vi "test Deployment Timing Channels.vi"(8 "error in":errorcluster, 11 "TestCase in":refnum<class "Deployment.lvclass">) -> (0 "error out":errorcluster, 3 "TestCase out":refnum<class "Deployment.lvclass">)   [LabVIEW 2023, in "Deployment.lvclass"]
uses:
  Deployment.lvclass
  Deployment.lvclass/Deployment.ctl
  <vilib>/addons/_JKI Toolkits/VI Tester/TestCase.llb/TestCase.lvclass
  315b1c3a-44c8-49e8-b756-01f865c29b4a.vi
  <vilib>/NI/VeriStand Custom Device Testing Tools/VeriStandTestUtilities/VeriStandTestUtilities.lvlib
  Scripting/Ballard MIL-STD-1553 Scripting.lvlib
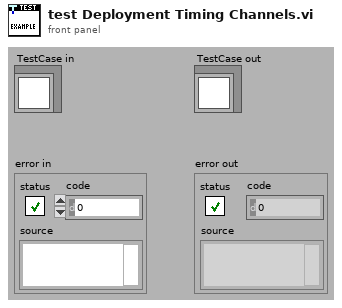
[diagram p1: front panel]
types:
  T1 = cluster{"Hardware File":path, "Parameters File":path}
  T2 = typedef "Custom Device API.lvlib/Custom Device Item Ref.ctl" = u64
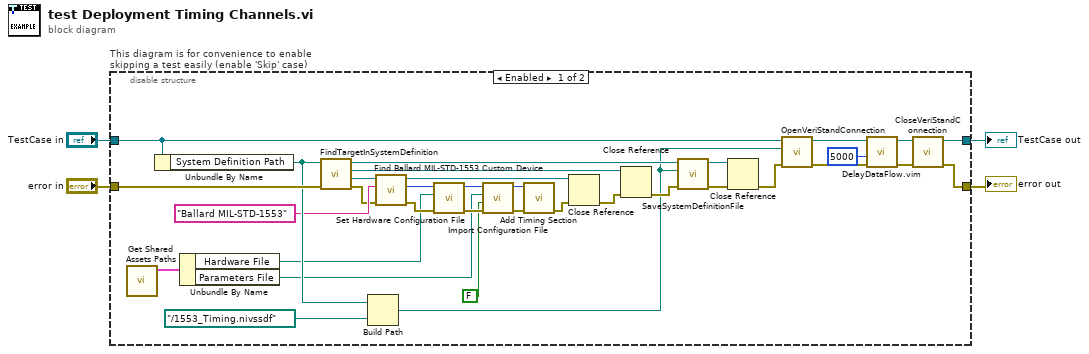
[diagram p0: block diagram]
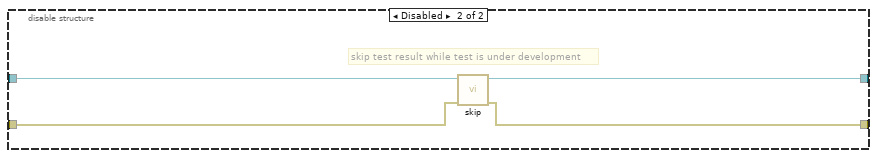
[diagram p2: hidden frame]
diagram:
  n1 = disable-structure "This diagram is for convenience to enable skipping a test easily (enable 'Skip' case)" shown="Enabled" {
    disable-tunnel: "TestCase in" -> [w31 w41]
    disable-tunnel: [w32 w39] -> w1
    disable-tunnel: [w34 w40] -> w3
    disable-tunnel: "error in" -> [w30 w38]
    frame Enabled {
      n2 = call "Get Shared Assets Paths.vi"() -> ("BC and RTs"=w8:T1)  [unwired: 9 in, 2 out]
      n3 = Unbundle By Name(w31) -> ("System Definition Path"=w28:path)
      n4 = Unbundle By Name(w8) -> ("Hardware File"=w10:path, "Parameters File"=w9:path)
      n5 = call <vilib>:"FindTargetInSystemDefinition.vi"("error in"=w30, "system definition path"=w28) -> ("error out"=w17:errorcluster, "Target"=w20:refnum<k24>, "Root"=w23:refnum<k24>, "System Definition"=w29:refnum<k24>)  [unwired: 6 in]
      n6 = Build Path(base path=w28, name or relative path=path "../1553_Timing.nivssdf") -> (appended path=w16:path)
      n7 = call "Find Ballard MIL-STD-1553 Custom Device.vi"("error in"=w17, "name"="Ballard MIL-STD-1553", "target in"=w20) -> ("error out"=w14:errorcluster, "Ballard MIL-STD 1553 custom device"=w13:T2, "target out"=w18:refnum<k24>)  [unwired: 5 in, 1 out]
      n8 = call "Set Hardware Configuration File.vi"("error in"=w14, "hardware configuration file path"=w10, "Ballard MIL-STD 1553 custom device in"=w13) -> ("error out"=w11:errorcluster, "Ballard MIL-STD 1553 custom device out"=w12:T2)  [unwired: 7 in]
      n9 = call "Import Configuration File.vi"("error in"=w11, "create Tx/Rx folders for subaddresses?"=FALSE, "parameters configuration file path"=w9, "Ballard MIL-STD 1553 custom device in"=w12) -> ("error out"=w15:errorcluster, "Ballard MIL-STD 1553 custom device out"=w6:T2)  [unwired: 6 in]
      n10 = call "Add Timing Section.vi"("error in"=w15, "custom device in"=w6) -> ("error out"=w7:errorcluster)  [unwired: 7 in, 2 out]
      n11 = Close Reference(reference=w18, error in (no error)=w7) -> (error out=w21:errorcluster)
      n12 = Close Reference(reference=w23, error in (no error)=w21) -> (error out=w22:errorcluster)
      n13 = call <vilib>:"SaveSystemDefinitionFile.vi"("error in (no error)"=w22, "System Definition File in"=w16, "System Definition Reference in"=w29) -> ("error out"=w25:errorcluster, "System Definition Reference out"=w26:refnum<k24>)  [unwired: 7 in]
      n14 = Close Reference(reference=w26, error in (no error)=w25) -> (error out=w24:errorcluster)
      n15 = call-dynamic "OpenVeriStandConnection.vi"("error in (no error)"=w24, "System Definition File"=w16, "VeriStand Test Case in"=w31) -> ("error out"=w37:errorcluster, "VeriStand Test Case out"=w33:refnum<class "Deployment.lvclass">)  [unwired: 6 in, 1 out]
      n16 = call "DelayDataFlow.vim"("value in"=w37, "milliseconds to wait"=u32 5000) -> ("value out"=w35:errorcluster)  [unwired: 2 in, 1 out]
      n17 = call-dynamic "CloseVeriStandConnection.vi"("error in (no error)"=w35, "VeriStand Test Case in"=w33) -> ("error out"=w34:errorcluster, "VeriStand Test Case out"=w32:refnum<class "Deployment.lvclass">)  [unwired: 8 in]
    }
    frame Disabled {
      # "skip test result while test is under development"
      n18 = call <vilib>:"skip.vi"("error in (no error)"=w38, "TestCase in"=w41) -> ("error out"=w40:errorcluster, "TestCase out"=w39:refnum<class "Deployment.lvclass">)  [unwired: 8 in]
    }
  }
  "error out" <- w3
  "TestCase out" <- w1
